vi "rawcdc_protocol_2_wSubVIch.vi"() -> ()   [LabVIEW 2024]
doc: "This example performs writes and reads on a serial port, as directed by the user. You can press the Write and Read buttons, and change the Read Count, while the example is running.\n\nThe parameters set for the serial port must match the parameters of the connected instrument or device. In this example, the Read Count parameter specifies the number of bytes that the serial port reads. If there were more bytes at the port than the specified number, those bytes would not be read. If there were less bytes at the port than the specified number, you would receive a timeout error.\n\nThis example expands upon the flow control options for XON and XOFF, allowing the user to choose those control characters. Also, the user can enable or disable a termination character. Some devices require a termination character in order to identify the end of command strings. Some devices send a termination character to signify the end of data to be read. This example shows how you can end the Read operation once a termination character is detected in the buffer and/or append a termination character at the end of the Write data."
panel:
  out "size(s)":i32[](array[numeric])
  out "Waveform Chart":dbl[][](graph)
  in  "Command List":string="stop\nencode 0\nslist 0 0\nslist 1 1\nsrate 6000\nps 2\ndec 1\ndeca 3\nnop\n"
  in  "Stop":bool
  in  "2108 CDC Virtual COM":refnum<visa-resource-name>="COM10"
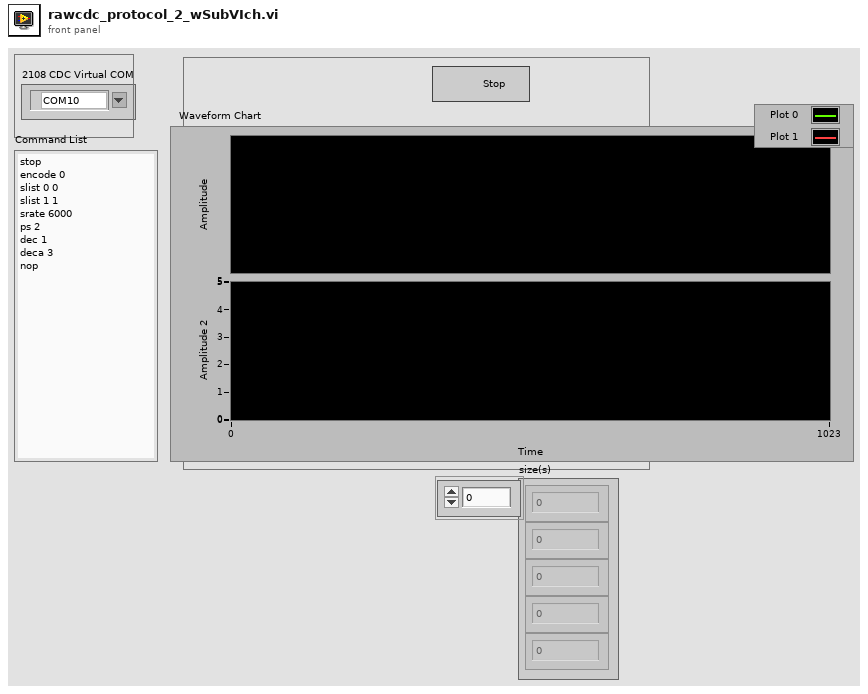
[diagram p1: front panel]
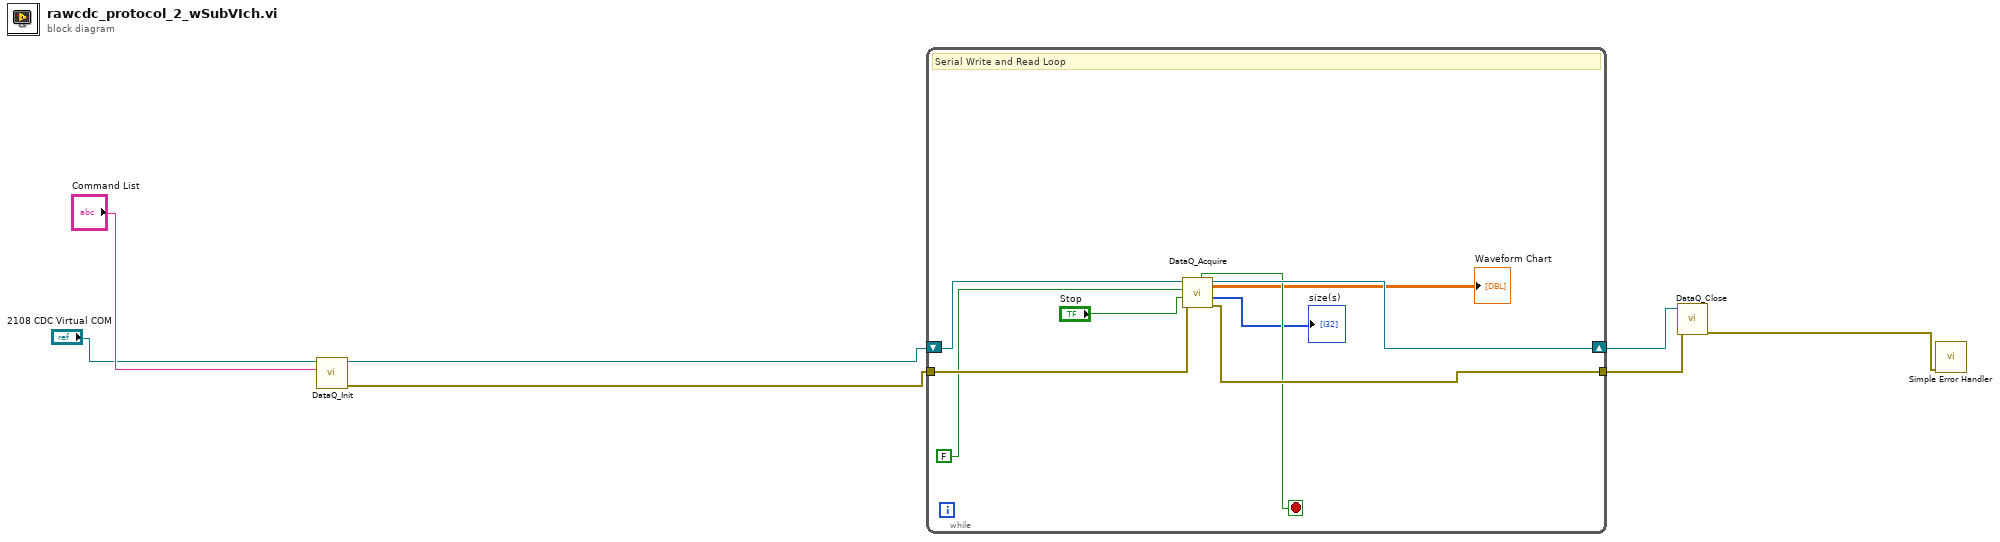
[diagram p0: block diagram]
diagram:
  n1 = call "DataQ_Init.vi"("Command List"="Command List", "VISA Refnum in"="2108 CDC Virtual COM") -> ("error out"=w1:errorcluster, "VISA Refnum out"=w2:refnum<visa-resource-name>)  [unwired: 8 in]
  n2 = while {
    shift-right: [w16] -> w4
    shift-left: w2 -> [w13]
    tunnel: w1 -> [w12]
    tunnel: [w15] -> w3
    stop <- w14 stop-if-true
    # "Serial Write and Read Loop"
    n3 = call "DataQ_Acquire.vi"("error in (no error)"=w12, "Stop in"="Stop", "Boolean"=FALSE, "VISA Refnum in"=w13) -> ("error out"=w15:errorcluster, "size(s)"=→"size(s)":i32[], "Array"=→"Waveform Chart":dbl[][], "VISA Refnum out"=w16:refnum<visa-resource-name>, "Stop out"=w14:bool)  [unwired: 3 in]
  }
  n4 = call "DataQ_Close.vi"("error in (no error)"=w3, "VISA Refnum in"=w4) -> ("error out"=w7:errorcluster)  [unwired: 9 in]
  n5 = call <vilib>:"Simple Error Handler.vi"("error in (no error)"=w7) -> ()  [unwired: 1 in, 8 out]
